vi "Connect Plugin.vi"(6 "Server Certificate File (.crt)":path, 8 "error in (no error)":errorcluster, 9 "VI Reference":refnum<vi>, 10 "Address":string, 11 "CIF_UI in":refnum<class "CIF_Plugin_UI.lvclass">) -> (0 "error out":errorcluster, 3 "CIF_UI out":refnum<class "CIF_Plugin_UI.lvclass">)   [LabVIEW 2021, in "CIF_Plugin_UI.lvclass"]
uses:
  CIF_Plugin_UI.lvclass
  D:/dev/CIF-LVCore/src/CIFUI/CIF_UI.lvclass
  CIFCore/Common/Typedef/Errors.ctl
  CIFUI/Typedef/Plugin Connections.ctl
  <vilib>/gRPC/LabVIEW gRPC Library/Shared/grpcId.ctl
  CIFPluginManager/CIFPluginManager/gRPC/CIF_Manager_client/RPC Messages/cif_manager_PluginInfo.ctl
  CIFPluginManager/CIFPluginManager/gRPC/CIF_Manager_client/RPC Messages/cif_manager_PluginVersion.ctl
  CIFPluginManager/CIFPluginManager/gRPC/CIF_Manager_client/RPC Messages/cif_plugincore_StatusData.ctl
  CIFPluginManager/CIFPluginManager/gRPC/CIF_Manager_client/RPC Messages/cif_plugincore_StatusData_State.ctl
  CIFPluginManager/CIFPluginManager/gRPC/CIF_Manager_client/RPC Messages/cif_plugincore_TimingStatistics.ctl
  CIFPluginManager/CIFPluginManager/gRPC/CIF_Manager_client/RPC Messages/cif_plugincore_TimingStatsBasic.ctl
  CIFPluginManager/CIFPluginManager/gRPC/CIF_Manager_client/RPC Messages/cif_plugincore_FifoStatistics.ctl
  CIFPluginManager/CIFPluginManager/gRPC/CIF_Manager_client/RPC Messages/cif_plugincore_Error.ctl
  CIFPluginManager/CIFPluginManager/gRPC/CIF_Manager_client/RPC Messages/cif_plugincore_MonitorDoubles.ctl
  CIFPluginManager/CIFPluginManager/gRPC/CIF_Manager_client/RPC Messages/cif_plugincore_MonitorU64.ctl
  CIFPluginManager/CIFPluginManager/gRPC/CIF_Manager_client/RPC Messages/cif_plugincore_MonitorI64.ctl
  CIFUI/CIF_UI.lvclass/CIF_UI.ctl
  <vilib>/Utility/miscctls.llb/LVMapReplaceAction.ctl
  CIFUI/Accessors/Read Plugin Connection Map.vi
  CIFUI/Accessors/Write IP Address.vi
  CIFUI/Accessors/Write VI Reference.vi
  CIFUI/Accessors/Write Plugin Connection Map.vi
  CIFUI/Accessors/Write Connected.vi
  CIFCore/Common/Utilities/Append Error Location.vi
  CIFPluginManager/CIFPluginManager/gRPC/CIF_Manager_client/CIF_Manager_client.lvlib
  <vilib>/gRPC/LabVIEW gRPC Library/grpc-lvsupport-release.lvlib
  CIFUI/CIF_UI.lvclass
  CIFCore/Common/CIFCoreCommon.lvlib
  CIFCore/Grpc/CIFCoreWrapper/CIFCoreWrapper.lvlib
  Plugins/Template/Grpc/Template_wrapper/TemplateWrapper.lvlib
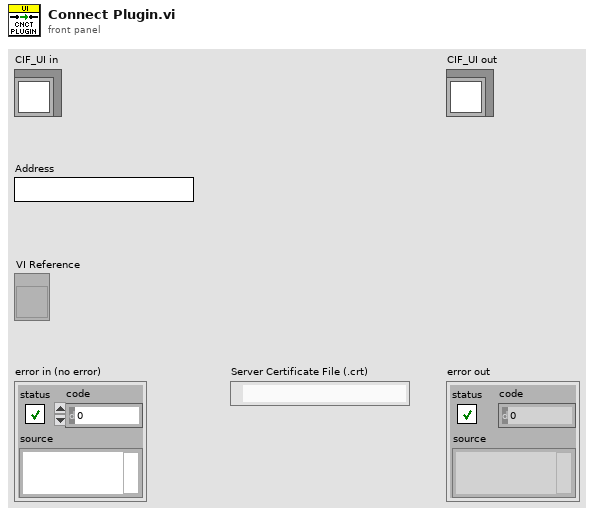
[diagram p1: front panel]
types:
  T1 = typedef "CIF_UI.lvclass/Plugin Connections.ctl" = cluster{"gRPC ID":T2, "Plugin info":T3}
  T2 = typedef "grpc-lvsupport-release.lvlib/grpcId.ctl" = u64
  T3 = typedef "CIF_Manager_client.lvlib/cif_manager_PluginInfo.ctl" = cluster{"plugin_name":string, "plugin_type":string, "grpc_port":i32, "plugin_version":T4, "status":T5}
  T4 = typedef "CIF_Manager_client.lvlib/cif_manager_PluginVersion.ctl" = cluster{"major_version":i32, "minor_version":i32, "fix_version":i32, "build_version":i32}
  T5 = typedef "CIF_Manager_client.lvlib/cif_plugincore_StatusData.ctl" = cluster{"state":T6, "timing_statistics":T7, "fifo_statistics":T9, "error":T10, "monitor_doubles":T11, "monitor_u64s":T12, "monitor_i64s":T13}
  T6 = typedef "CIF_Manager_client.lvlib/cif_plugincore_StatusData_State.ctl" = enum32{"NULL", "CREATING", "LISTENING", "RUNNING", "CLEANINGUP", "DESTROYING"}
  T7 = typedef "CIF_Manager_client.lvlib/cif_plugincore_TimingStatistics.ctl" = cluster{"period":T8, "wake_error":T8, "execute":T8, "housekeep":T8, "idle":T8}
  T8 = typedef "CIF_Manager_client.lvlib/cif_plugincore_TimingStatsBasic.ctl" = cluster{"max":i32, "min":i32}
  T9 = typedef "CIF_Manager_client.lvlib/cif_plugincore_FifoStatistics.ctl" = cluster{"from_t0":T8, "from_previous_plugin":T8, "output_error":T8}
  T10 = typedef "CIF_Manager_client.lvlib/cif_plugincore_Error.ctl" = cluster{"status":bool, "code":i32}
  T11 = typedef "CIF_Manager_client.lvlib/cif_plugincore_MonitorDoubles.ctl" = cluster{"double_1":dbl, "double_2":dbl, "double_3":dbl, "double_4":dbl}
  T12 = typedef "CIF_Manager_client.lvlib/cif_plugincore_MonitorU64.ctl" = cluster{"u64_1":u64, "u64_2":u64, "u64_3":u64, "u64_4":u64}
  T13 = typedef "CIF_Manager_client.lvlib/cif_plugincore_MonitorI64.ctl" = cluster{"i64_1":i64, "i64_2":i64, "i64_3":i64, "i64_4":i64}
  T14 = typedef "CIFCoreCommon.lvlib/Errors.ctl" = enum16{"Invalid Clock ID", "Long Sleep", "gRPC Server Not Found", "Config Parse", "Timestamp Wrap", "Delayed Execution", "Duplicate Channel", "Missing Channel", "Incorrect Type", "Flatten Error", "Unflatten Data", "Unique Name", "Plugin Not Found", "Plugin Type Not Found", "Plugin Version Not Found", "Manager Not Found", "Numerical Issue", "Time Jump", "Clock ID Match", "Channel Length", "Plugin Connection", "gRPC Server Connection"}
  T15 = typedef "LVMapReplaceAction.ctl" = enum32{"Modify Entry only if found", "Add or Modify Entry", "Delete Entry"}
  T16 = typedef "CIFCoreCommon.lvlib/Version.ctl" = cluster{"Major":i32, "Minor":i32, "Fix":i32, "Build":i32}
  T17 = typedef "CIF_UI.lvclass/Plugin Connection Map.ctl" = map{string, T1}
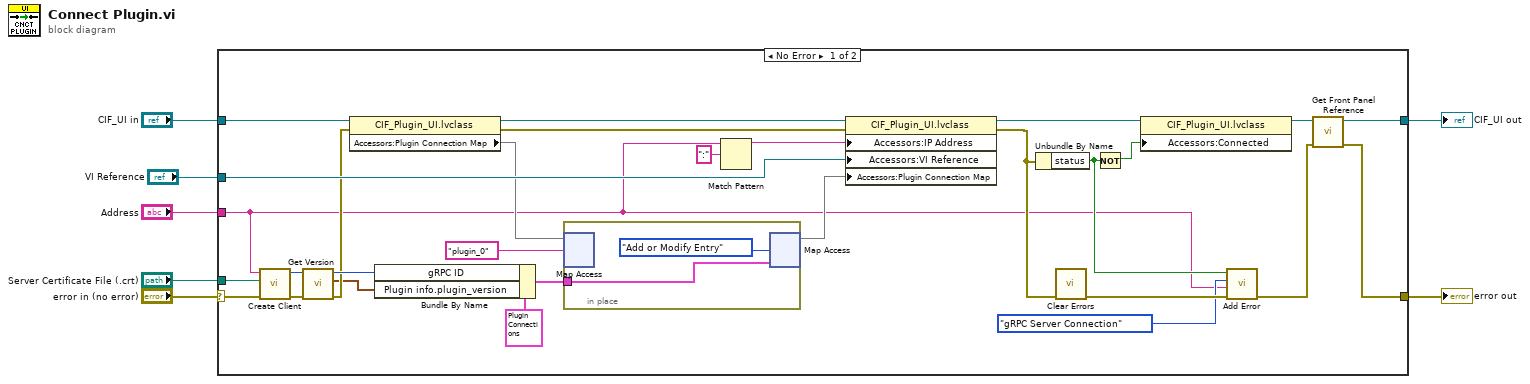
[diagram p0: block diagram]
diagram:
  n1 = case shown="No Error" "error in (no error)" {
    selector: "error in (no error)" -> [w11 w40]
    tunnel: [w14 w40] -> w6
    tunnel: [w13 w39] -> w4
    tunnel: "CIF_UI in" -> [w27 w39]
    tunnel: "Address" -> [w12 _]
    tunnel: "VI Reference" -> [w28 _]
    tunnel: "Server Certificate File (.crt)" -> [w10 _]
    frame No Error {
      n2 = call "Create Client.vi"("error in"=w11, "Server Certificate File (.crt)"=w10, "address"=w12) -> ("error out"=w9:errorcluster, "gRPC ID Out"=w8:T2)  [unwired: 7 in]
      n3 = call "Get Version.vi"("error in"=w9, "gRPC ID"=w8) -> ("error out"=w21:errorcluster, "Version"=w19:T16, "gRPC ID out"=w30:T2)  [unwired: 7 in]
      n4 = property class="CIF_Plugin_UI.lvclass"(reference=w27, error in=w21) -> (reference out=w26:refnum<class "CIF_Plugin_UI.lvclass">, error out=w20:errorcluster, "Accessors:Plugin Connection Map"=w25:T17)
      n5 = Bundle By Name(cluster=T1 {"gRPC ID"=0, "Plugin info"={"plugin_name"="", "plugin_type"="", "grpc_port"=0, "plugin_version"={"major_version"=0, "minor_version"=0, "fix_version"=0, "build_version"=0}, "status"={"state"=enum."NULL", "timing_statistics"={"period"={"max"=0, "min"=0}, "wake_error"={"max"=0, "min"=0}, "execute"={"max"=0, "min"=0}, "housekeep"={"max"=0, "min"=0}, "idle"={"max"=0, "min"=0}}, "fifo_statistics"={"from_t0"={"max"=0, "min"=0}, "from_previous_plugin"={"max"=0, "min"=0}, "output_error"={"max"=0, "min"=0}}, "error"={"status"=FALSE, "code"=0}, "monitor_doubles"={"double_1"=0.0, "double_2"=0.0, "double_3"=0.0, "double_4"=0.0}, "monitor_u64s"={"u64_1"=0, "u64_2"=0, "u64_3"=0, "u64_4"=0}, "monitor_i64s"={"i64_1"=0, "i64_2"=0, "i64_3"=0, "i64_4"=0}}}} ("value"), "gRPC ID"=w30, "Plugin info.plugin_version"=w19) -> (w23:T1)
      n6 = in-place {
        in-place-border: w23 -> [w38]
        n7 = in-place-map #1(w25, "plugin_0" ("key")) -> ()  [unwired: 1 in, 2 out]
        n8 = in-place-map #1(w38, LVMapReplaceAction."Add or Modify Entry" ("action")) -> (w22:T17)  [unwired: 2 out]
      }
      n9 = Match Pattern(string=w12, regular expression=":") -> (before substring=w29:string)  [unwired: 1 in, 3 out]
      n10 = property class="CIF_Plugin_UI.lvclass"(reference=w26, error in=w20, "Accessors:IP Address"=w29, "Accessors:VI Reference"=w28, "Accessors:Plugin Connection Map"=w22) -> (reference out=w18:refnum<class "CIF_Plugin_UI.lvclass">, error out=w16:errorcluster)
      n11 = Unbundle By Name(w16) -> ("status"=w33:bool)
      n12 = call <vilib>:"Clear Errors.vi"("error in (no error)"=w16) -> ("error out"=w35:errorcluster)  [unwired: 5 in, 1 out]
      n13 = Not(x=w33) -> (.not. x?=w17:bool)
      n14 = property class="CIF_Plugin_UI.lvclass"(reference=w18, "Accessors:Connected"=w17) -> (reference out=w15:refnum<class "CIF_Plugin_UI.lvclass">)  [unwired: 1 in, 1 out]
      n15 = call "Add Error.vi"("error in (no error)"=w35, "String to Append"=w12, "Error"=Errors."gRPC Server Connection", "Insert Error"=w33) -> ("error out"=w34:errorcluster)  [unwired: 7 in]
      n16 = call "Get Front Panel Reference.vi"("error in (no error)"=w34, "CIF_UI in"=w15) -> ("error out"=w14:errorcluster, "CIF_UI out"=w13:refnum<class "CIF_Plugin_UI.lvclass">)  [unwired: 8 in]
    }
    frame Error {
    }
  }
  "error out" <- w6
  "CIF_UI out" <- w4
